vi "CreateRenderer.vi"(8 "No Error":errorcluster, 10 "name (\"\": NULL)":string, 11 "window [SDL_Window *]":i64) -> (0 "error out":errorcluster, 3 "renderer [SDL_Renderer *]":i64)   [LabVIEW 2024, in "SDL3.lvlib" / "Render.lvlib"]
doc: "<B>Summary</B>\nCreate a 2D rendering context for a window.\n\n<B>Remarks</B>\nIf you want a specific renderer, you can specify its name here. A list of available renderers can be obtained by calling SDL_GetRenderDriver multiple times, with indices from 0 to SDL_GetNumRenderDrivers()-1. If you don't need a specific renderer, specify NULL and SDL will attempt to choose the best option for you, based on what is available on the user's system.\n\nBy default the rendering size matches the window size in pixels, but you can call SDL_SetRenderLogicalPresentation() to change the content size and scaling options.\n\n<B>Thread Safety</B>\nYou may only call this function from the main thread."
uses:
  Render.lvlib
  Error/Error.lvlib
  Lib/SDL3-32.dll
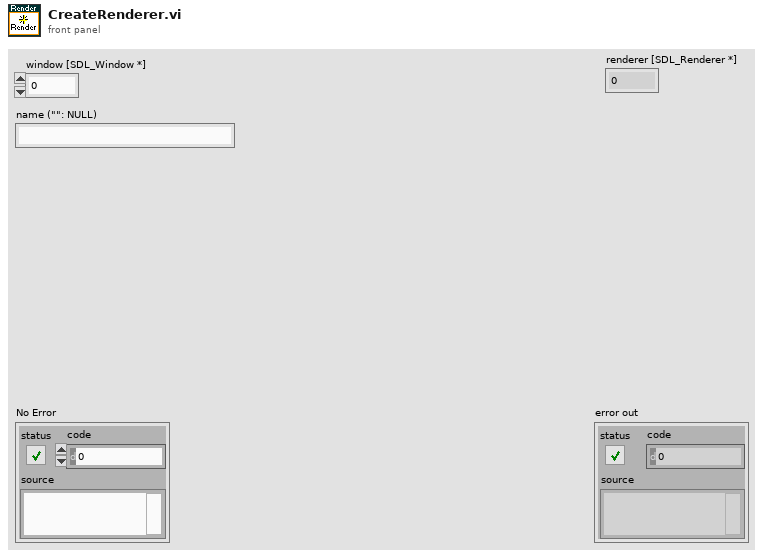
[diagram p1: front panel]
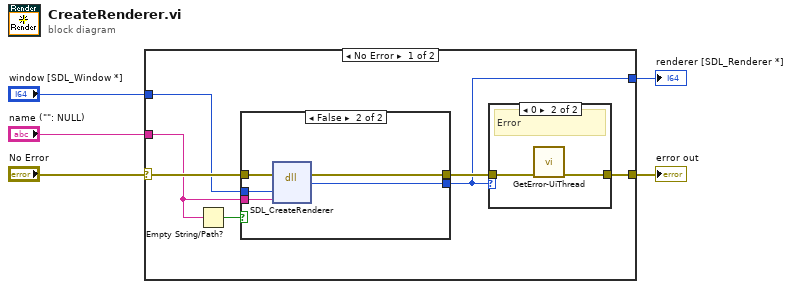
[diagram p0: block diagram]
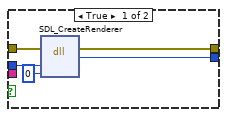
[diagram p2: hidden frame]
diagram:
  n1 = case shown="No Error" "No Error" {
    selector: "No Error" -> [w12 w26]
    tunnel: [w10 w26] -> w4
    tunnel: "name (\"\": NULL)" -> [w7 _]
    tunnel: [w9 _] -> w2
    tunnel: "window [SDL_Window *]" -> [w8 _]
    frame No Error {
      n2 = Empty String/Path?(string/path=w7) -> (empty?=w6:bool)
      n3 = case shown="False" w6 {
        tunnel: w12 -> [w17 w22]
        tunnel: [w16 w21] -> w11
        tunnel: w7 -> [_ w20]
        tunnel: [w15 w19] -> w9
        tunnel: w8 -> [w14 w18]
        frame True {
          n4 = dll-call lib="C:/Users/Thomas/Documents/Projects/LV-SDL3/Lib/SDL3-*.*" fn="SDL_CreateRenderer"(error in=w17, "window"=w14, "title"=i64 0) -> (error out=w16:errorcluster, "return type"=w15:i64)  [unwired: 4 in, 1 out]
        }
        frame False {
          n5 = dll-call lib="C:/Users/Thomas/Documents/Projects/LV-SDL3/Lib/SDL3-*.*" fn="SDL_CreateRenderer"(error in=w22, "window"=w18, "title"=w20) -> (error out=w21:errorcluster, "return type"=w19:i64)  [unwired: 4 in, 1 out]
        }
      }
      n6 = case shown="0" w9 {
        tunnel: w11 -> [w23 w25]
        tunnel: [w23 w24] -> w10
        frame Default {
          # "Ok"
        }
        frame 0 {
          # "Error"
          n7 = call "GetError-UiThread.vi"("No Error"=w25) -> ("error out"=w24:errorcluster)  [unwired: 10 in]
        }
      }
    }
    frame Error {
    }
  }
  "error out" <- w4
  "renderer [SDL_Renderer *]" <- w2
